vi "Kalman Filter - Update Step.vi"(8 "Dynamical System Matrices In":T1, 9 "Observations":T2, 10 "Old Covariance":T2, 11 "Old State":T2) -> (0 "Dynamical System Matrices Out":T1, 2 "Updated Covariance":T2, 3 "Updated State":T2)   [LabVIEW 2020]
uses:
  ctl/Dynamical System Matrices.ctl
  <vilib>/Analysis/Matrix/Datatypes/RealMatrix.ctl
  <vilib>/Analysis/Matrix/NI_Matrix.lvlib
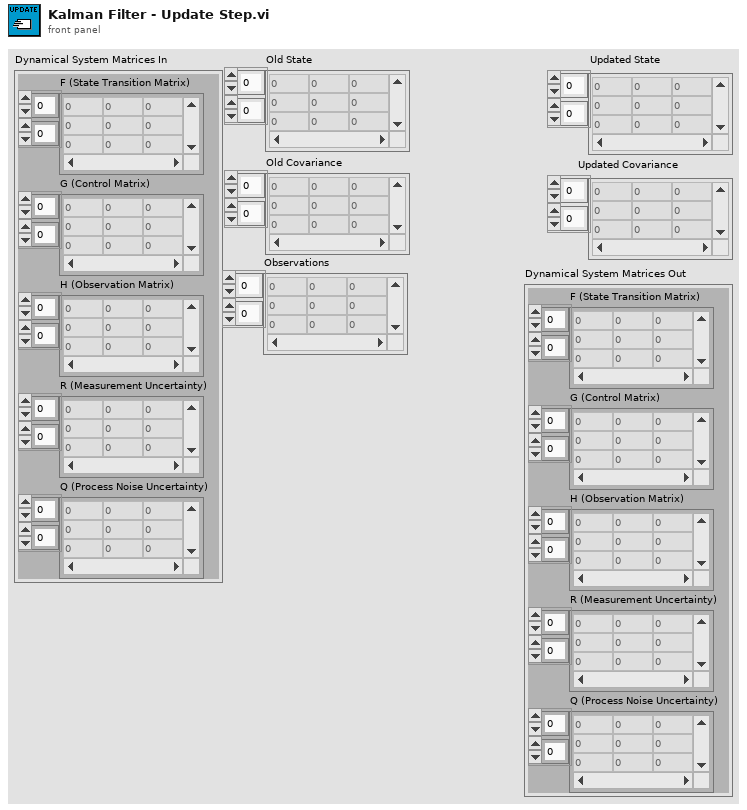
[diagram p1: front panel]
types:
  T1 = typedef "Dynamical System Matrices.ctl" = cluster{"F (State Transition Matrix)":T2, "G (Control Matrix)":T2, "H (Observation Matrix)":T2, "R (Measurement Uncertainty)":T2, "Q (Process Noise Uncertainty)":T2}
  T2 = typedef "NI_Matrix.lvlib/RealMatrix.ctl" = dbl[][]
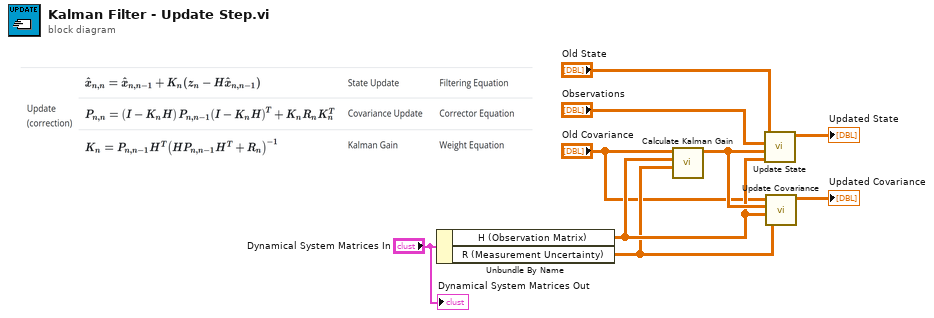
[diagram p0: block diagram]
diagram:
  n1 = Unbundle By Name("Dynamical System Matrices In") -> ("H (Observation Matrix)"=w8:T2, "R (Measurement Uncertainty)"=w7:T2)
  n2 = call "Calculate Kalman Gain.vi"("R"=w7, "H"=w8, "Covariance"="Old Covariance") -> ("Kalman Gain"=w9:T2)  [unwired: 8 in]
  n3 = call "Update State.vi"("H"=w8, "K"=w9, "Observations"="Observations", "Old State"="Old State") -> ("Updated State"=→"Updated State":T2)  [unwired: 7 in]
  n4 = call "Update Covariance.vi"("R"=w7, "H"=w8, "K"=w9, "Old Covariance"="Old Covariance") -> ("Updated Covariance"=→"Updated Covariance":T2)  [unwired: 7 in]
  "Dynamical System Matrices Out" <- "Dynamical System Matrices In"
